vi "RungeKuttaTimeVarying_Rk4_Mat_T_Y.vi"(5 "Func_T_Y_Extra":refnum<vi>, 7 "PassedData":variant, 8 "dT_Seconds":dbl, 10 "Y":T1, 11 "T":dbl) -> (0 "Error":bool, 3 "OUTPUT":T1)   [LabVIEW 2019, in "Trajectory_Library.lvlib"]
doc: "Performs 4th order Runge-Kutta integration of dx/dt = f( t, matrix y) for dt.\n\nInputs:\n - Func_T_Y_Extra -- A strictly typed LabVIEW reference to a function to integrate as a function of matrix T, Y, and the extra passed data\n - PassedData -- This is a variant that can be used to pass additional data to the function if needed. The data must be packed into the variant in the specific way expected by the function.\n - T -- The initial value of T\n - Y -- The initial value of Y.\n - dT -- The time over which to integrate\n\nOutputs:\n - OUTPUT -- The integration of dx/dt = f(t, y) for dt.\n - Error -- If TRUE, an error occured."
uses:
  Trajectory_Library.lvlib
  <vilib>/Analysis/Matrix/Datatypes/RealMatrix.ctl
  <vilib>/Analysis/Matrix/Numeric/Multiply/Multiply - RM,R.vi
  <vilib>/Analysis/Matrix/Numeric/Add/Add - RM,RM.vi
  <vilib>/Analysis/Matrix/NI_Matrix.lvlib
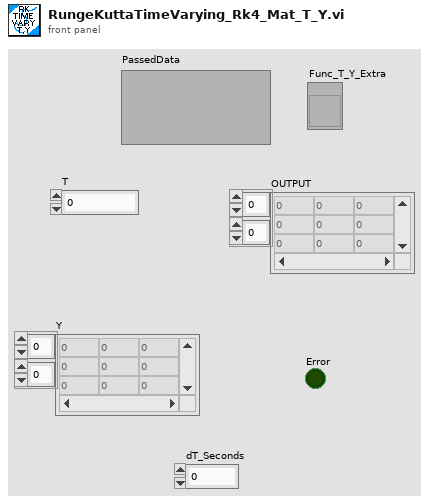
[diagram p1: front panel]
types:
  T1 = typedef "NI_Matrix.lvlib/RealMatrix.ctl" = dbl[][]
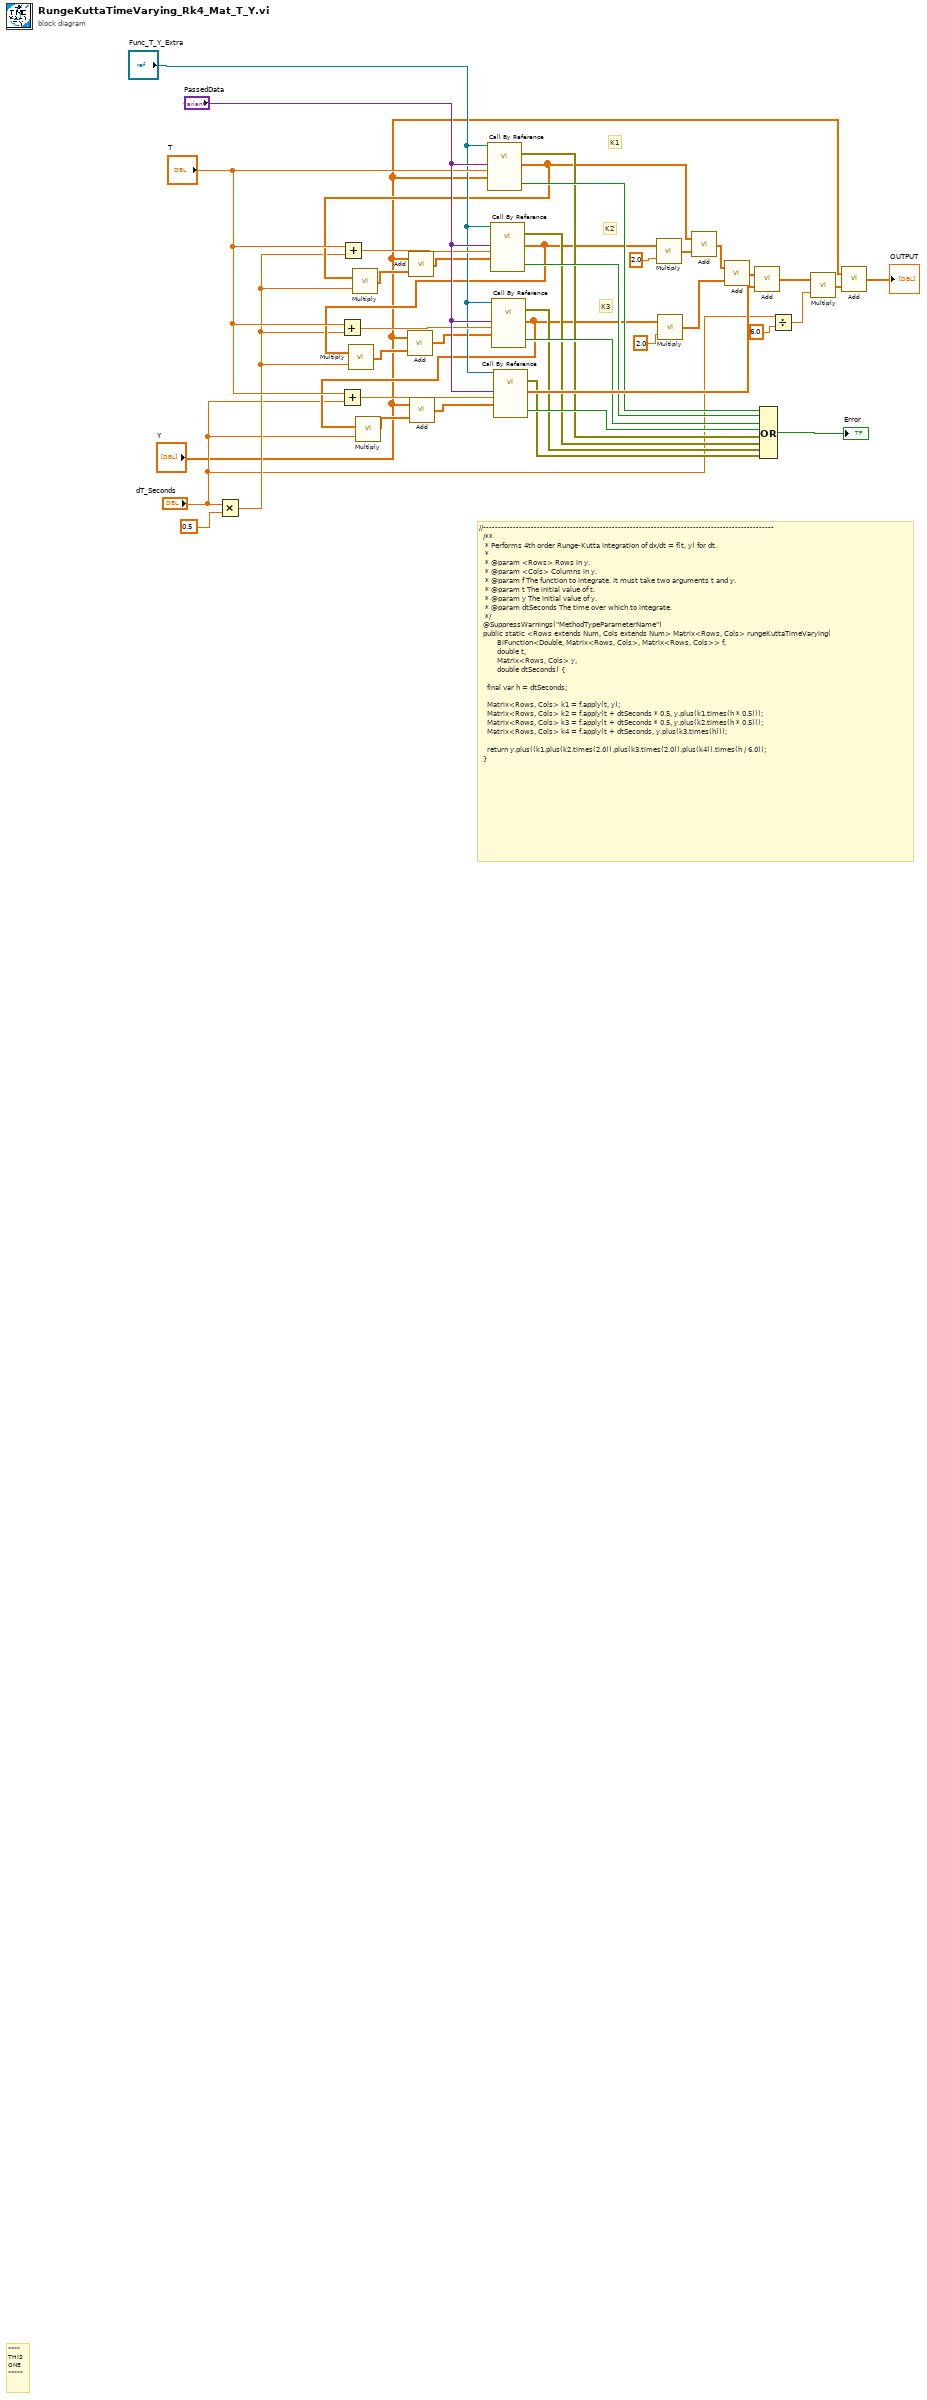
[diagram p0: block diagram]
diagram:
  # "//-------------------------------------------------------------------------------------------------\n  /**\n   * Performs 4th order Runge-Kutta integration of dx/dt = f(t, y) for dt.\n   *\n   * @param <Rows> Rows in y.\n   * @param <Cols> Columns in y.\n   * @param f The function to integrate. It must take two arguments t and y.\n   * @param t The initial value of t.\n   * @param y The initial value of y.\n   * @param dtSeconds The time over which to integrate.\n   */\n  @SuppressWarnings(\"MethodTypeParameterName\")\n  public static <Rows extends Num, Cols extends Num> Matrix<Rows, Cols> rungeKuttaTimeVarying(\n      \t\t\tBiFunction<Double, Matrix<Rows, Cols>, Matrix<Rows, Cols>> f,\n      \t\t\tdouble t,\n      \t\t\tMatrix<Rows, Cols> y,\n      \t\t\tdouble dtSeconds) {\n\n    final var h = dtSeconds;\n\n    Matrix<Rows, Cols> k1 = f.apply(t, y);\n    Matrix<Rows, Cols> k2 = f.apply(t + dtSeconds * 0.5, y.plus(k1.times(h * 0.5)));\n    Matrix<Rows, Cols> k3 = f.apply(t + dtSeconds * 0.5, y.plus(k2.times(h * 0.5)));\n    Matrix<Rows, Cols> k4 = f.apply(t + dtSeconds, y.plus(k3.times(h)));\n\n    return y.plus((k1.plus(k2.times(2.0)).plus(k3.times(2.0)).plus(k4)).times(h / 6.0));\n  }"
  # "K3"
  # "K2"
  # "K1"
  # "****\nTHIS\nONE\n*****"
  n1 = Multiply(x="dT_Seconds", y=0.5) -> (x*y=w3:dbl)
  n2 = Add ("Add.vi")(x="T", y=w3) -> (x+y=w25:dbl)
  n3 = Add ("Add.vi")(x="T", y="dT_Seconds") -> (x+y=w24:dbl)
  n4 = Add ("Add.vi")(x="T", y=w3) -> (x+y=w26:dbl)
  n5 = call-by-ref "?"(reference="Func_T_Y_Extra", "Y"="Y", "T"="T", "Variant"="PassedData") -> (error out=w17:errorcluster, "Error"=w32:bool, "Output"=w6:T1)  [unwired: 8 in, 1 out]
  n6 = call-poly <vilib>:"Multiply.vi"("Real Scalar c"=w3, "Real Matrix A"=w6) -> ("A * c"=w12:T1)
  n7 = call-poly <vilib>:"Add.vi"("Real Matrix B"=w12, "Real Matrix A"="Y") -> ("A + B"=w9:T1)
  n8 = call-by-ref "?"(reference="Func_T_Y_Extra", "Y"=w9, "T"=w26, "Variant"="PassedData") -> (error out=w16:errorcluster, "Error"=w31:bool, "Output"=w5:T1)  [unwired: 8 in, 1 out]
  n9 = call-poly <vilib>:"Multiply.vi"("Real Scalar c"=w3, "Real Matrix A"=w5) -> ("A * c"=w11:T1)
  n10 = call-poly <vilib>:"Add.vi"("Real Matrix B"=w11, "Real Matrix A"="Y") -> ("A + B"=w8:T1)
  n11 = call-by-ref "?"(reference="Func_T_Y_Extra", "Y"=w8, "T"=w25, "Variant"="PassedData") -> (error out=w15:errorcluster, "Error"=w30:bool, "Output"=w4:T1)  [unwired: 8 in, 1 out]
  n12 = call-poly <vilib>:"Multiply.vi"("Real Scalar c"="dT_Seconds", "Real Matrix A"=w4) -> ("A * c"=w10:T1)
  n13 = call-poly <vilib>:"Add.vi"("Real Matrix B"=w10, "Real Matrix A"="Y") -> ("A + B"=w7:T1)
  n14 = call-by-ref "?"(reference="Func_T_Y_Extra", "Y"=w7, "T"=w24, "Variant"="PassedData") -> (error out=w14:errorcluster, "Error"=w29:bool, "Output"=w33:T1)  [unwired: 8 in, 1 out]
  n15 = call-poly <vilib>:"Multiply.vi"("Real Scalar c"=2.0, "Real Matrix A"=w5) -> ("A * c"=w37:T1)
  n16 = call-poly <vilib>:"Multiply.vi"("Real Scalar c"=2.0, "Real Matrix A"=w4) -> ("A * c"=w35:T1)
  n17 = call-poly <vilib>:"Add.vi"("Real Matrix B"=w37, "Real Matrix A"=w6) -> ("A + B"=w36:T1)
  n18 = call-poly <vilib>:"Add.vi"("Real Matrix B"=w35, "Real Matrix A"=w36) -> ("A + B"=w34:T1)
  n19 = call-poly <vilib>:"Add.vi"("Real Matrix B"=w33, "Real Matrix A"=w34) -> ("A + B"=w23:T1)
  n20 = Compound Arithmetic op=OR(w32, w31, w30, w29, w17, w16, w15, w14) -> (→"Error":bool)
  n21 = Divide(x="dT_Seconds", y=6.0) -> (x/y=w21:dbl)
  n22 = call-poly <vilib>:"Multiply.vi"("Real Scalar c"=w21, "Real Matrix A"=w23) -> ("A * c"=w20:T1)
  n23 = call-poly <vilib>:"Add.vi"("Real Matrix B"=w20, "Real Matrix A"="Y") -> ("A + B"=→"OUTPUT":T1)
